vi "Read Name.vi"(11 "RetentionPolicy in":refnum<class "RetentionPolicy.lvclass">) -> (2 "Name":string, 3 "RetentionPolicy out":refnum<class "RetentionPolicy.lvclass">)   [LabVIEW 2018, in "InfluxDB Client.lvlib" / "RetentionPolicy.lvclass"]
uses:
  RetentionPolicy.lvclass
  RetentionPolicy.lvclass/RetentionPolicy.ctl
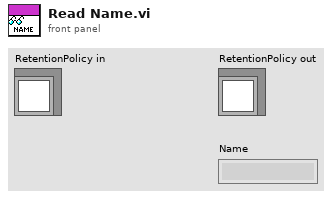
[diagram p1: front panel]
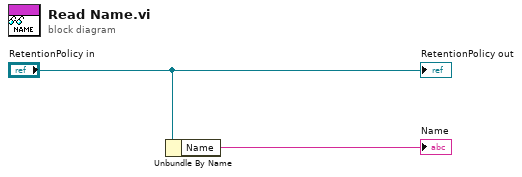
[diagram p0: block diagram]
diagram:
  n1 = Unbundle By Name("RetentionPolicy in") -> ("Name"=→"Name":string)
  "RetentionPolicy out" <- "RetentionPolicy in"
